vi "3 Tap 12-Bit.vi"() -> (0 "Pixels":T1)   [LabVIEW 2013]
uses:
  <vilib>/rvi/eio/common/nirviEmuTemplateMethod_errors.vi
  <vilib>/eio/EIONode/EIONode.xnode
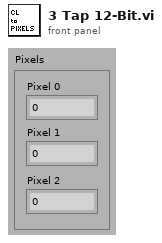
[diagram p1: front panel]
types:
  T1 = cluster{"Pixel 0":u16, "Pixel 1":u16, "Pixel 2":u16}
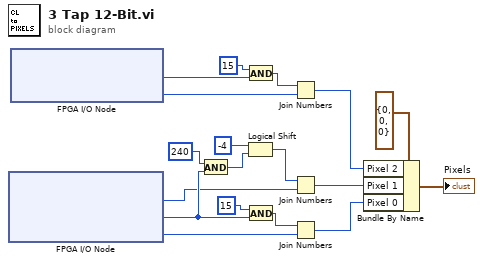
[diagram p0: block diagram]
diagram:
  n1 = xnode "FPGA I/O Node"() -> ("IO Module\\CL Port C"=w10:u8, "IO Module\\CL Port B"=w12:u8, "IO Module\\CL Port A"=w11:u8)  [unwired: 3 in, 3 out]
  n2 = xnode "FPGA I/O Node"() -> ("IO Module\\CL Port F"=w3:u8, "IO Module\\CL Port E"=w2:u8)  [unwired: 2 in, 2 out]
  n3 = And(x=u8 240 ("hi"), y=w12) -> (x .and. y?=w15:u8)
  n4 = Logical Shift(y=i8 -4, x=w15) -> (x << y=w13:u8)
  n5 = And(x=u8 15 ("hi"), y=w3) -> (x .and. y?=w5:u8)
  n6 = And(x=u8 15 ("hi"), y=w12) -> (x .and. y?=w17:u8)
  n7 = Join Numbers(hi=w5, lo=w2) -> ((hi.lo)=w1:u16)
  n8 = Join Numbers(hi=w13, lo=w10) -> ((hi.lo)=w8:u16)
  n9 = Join Numbers(hi=w17, lo=w11) -> ((hi.lo)=w9:u16)
  n10 = Bundle By Name(cluster=T1 {"Pixel 0"=0, "Pixel 1"=0, "Pixel 2"=0} ("PixelData"), "Pixel 2"=w1, "Pixel 1"=w8, "Pixel 0"=w9) -> (→"Pixels":T1)
